vi "Maxi Gauge-RW Set Point.vi"(0 "VISA-Ressource in":refnum<visa-resource-name>, 1 "Node address":i8=-1 min=-1 max=31 step=1, 2 "W/R":bool, 5 "Relay Nr.:":i32(ring) items=["Relay A", "Relay B", "Relay C", "Relay D", "Relay E", "Relay F"], 7 "Control Sensor :":i32(ring) items=["sensor 1", "sensor 2", "sensor 3", "sensor 4", "sensor 5", "sensor 6"], 9 "Setpoint low":dbl=1e-13 min=1e-13 max=41000.0 format="%.2e", 11 "Fehler (Eingang)":errorcluster, 12 "Setpoint high":dbl=1e-13 min=1e-13 max=41000.0 format="%.2e") -> (4 "VISA-Ressource out":refnum<visa-resource-name>, 6 "Get Control Sensor:":i32(ring) items=["sensor 1", "sensor 2", "sensor 3", "sensor 4", "sensor 5", "sensor 6"], 8 "Get Setpoint low":dbl=1e-13 min=1e-13 max=41000.0 format="%.2e", 10 "Get Setpoint high":dbl=1e-13 min=1e-13 max=41000.0 format="%.2e", 15 "Fehler (Ausgang)":errorcluster)   [LabVIEW 2012, in "Maxi Gauge.lvlib"]
uses:
  Maxi Gauge.lvlib
panel:
  # "mbar"
  # "mbar"
  # "mbar"
  # "mbar"
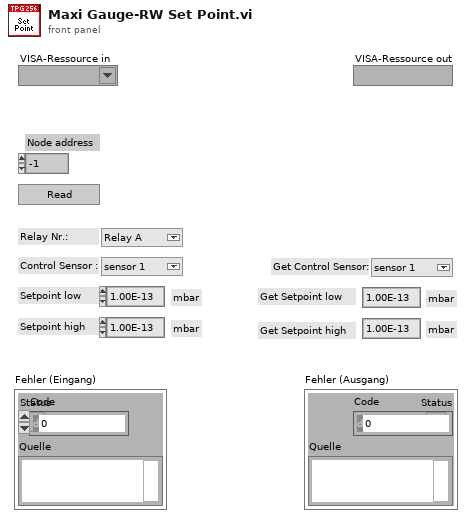
[diagram p1: front panel]
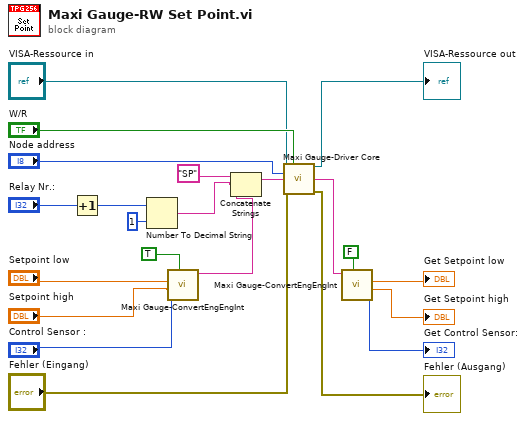
[diagram p0: block diagram]
diagram:
  n1 = Increment(x="Relay Nr.:") -> (x+1=w14:i32)
  n2 = Number To Decimal String(number=w14, width (-)=i16 1) -> (decimal integer string=w6:string)
  n3 = call "Maxi Gauge-ConvertEngEngInt.vi"("W/R [W: Int in; Str out ]"=TRUE, "Integer1 in"="Control Sensor :", "Eng2 in"="Setpoint high", "Eng1 in"="Setpoint low") -> ("String out"=w10:string)  [unwired: 4 in, 3 out]
  n4 = Concatenate Strings("SP" ("Command"), w6, w10) -> (w5:string)
  n5 = call "Maxi Gauge-Driver Core.vi"("VISA-Ressource in"="VISA-Ressource in", "Write/Read"="W/R", "Node address"="Node address", "Command"=w5, "Fehler (Eingang)"="Fehler (Eingang)") -> ("VISA-Ressource out"=→"VISA-Ressource out":refnum<visa-resource-name>, "String Out"=w8:string, "Fehler (Ausgang)"=→"Fehler (Ausgang)":errorcluster)  [unwired: 8 in]
  n6 = call "Maxi Gauge-ConvertEngEngInt.vi"("W/R [W: Int in; Str out ]"=FALSE, "String in"=w8) -> ("Integer1 out"=→"Get Control Sensor:":u8, "Eng2 out"=→"Get Setpoint high":dbl, "Eng1 out"=→"Get Setpoint low":dbl)  [unwired: 6 in, 1 out]
